vi "LSMcontroller_v57.vi"() -> ()   [LabVIEW 2015] (continued)
                      frame "X-Y Image", Default {
                        n4025 = local read "Sampling rate"() -> (w685:dbl)
                      }
                      frame "Timetrace" {
                        n4026 = local read "srateAODOtt"() -> (w686:dbl)
                      }
                    }
                    n4027 = call "waveformsAObuffer.vi"("command"="get") -> ("AO wf out"=w684:waveform(dbl)[])  [unwired: 1 in]
                    n4028 = Build Array (concatenate)(w671, w669) -> (w675:digitalwaveform[])
                    n4029 = call "correctwaveformsizetemp.vi"("new sampling frequency (Hz)"=w665, "start"=FALSE, "reference waveforms to"=w676, "Analog waveforms in"=w684, "stop"=FALSE, "Digital waveforms in"=w675) -> ("analog wf out"=w679:waveform(dbl)[], "Digital wf out"=w677:digitalwaveform[], "measpoints"=w667:i32)
                    n4030 = local write "Analog Lines Plot"(w679) -> ()
                    n4031 = call "GetNumCamFramesv2.vi"("Digital Waveform Graph"=w677) -> ("Numeric"=w678:i32)  [unwired: 10 in]
                    n4032 = local write "Digital Lines Plot"(w677) -> ()
                    n4033 = call "waveformsAObuffer.vi"("AO wf in"=w679, "command"="set") -> ()  [unwired: 1 out]
                    n4034 = call "waveformsDObuffer.vi"("DO wf in"=w677, "command"="set") -> ()  [unwired: 1 out]
                    n4035 = local write "Total Camera Frames"(w678) -> ()
                    n4036 = local read "wavdet"() -> (w668:bool)
                    n4037 = case shown="True" w668 {
                      tunnel: w667 -> [_ w687]
                      frame False {
                      }
                      frame True {
                        n4038 = local write "# of frames"(w687) -> ()
                      }
                    }
                  }
                  frame #7 {
                    w693 = FALSE ("addAO")
                    n4039 = local read "finite samples"() -> (w694:bool)
                    n4040 = local read "continuous"() -> (w695:bool)
                    n4041 = local read "wavdet"() -> (w696:bool)
                    n4042 = call "2pparameters.vi"("command"="get") -> ("params out"=w699:T12)  [unwired: 1 in]
                    n4043 = Bundle By Name(cluster=w699, "finite"=w694, "cont"=w695, "wavdet"=w696) -> (w697:T12)
                    n4044 = call "2pparameters.vi"("Params in"=w697, "command"="set") -> ()  [unwired: 1 out]
                    n4045 = local write "addDO"(w693) -> ()
                    n4046 = property on="Add DO wave" class="Bool (strict)"("Val(Sgnl)"=w693) -> ()  [unwired: 2 in, 2 out]
                  }
                }
              }
            }
          }
          event "DO channels": Value Change {
            n4047 = event-data() -> ()  [unwired: 1 in, 6 out]
            n4048 = local read "DO channels"() -> (w703:u16)
            n4049 = call "2pparameters.vi"("command"="get") -> ("params out"=w705:T12)  [unwired: 1 in]
            n4050 = Unbundle By Name(w705) -> ("aDO"=w704:u32[])
            n4051 = Search 1D Array(1D array=w704, element=w703) -> (index of element=w702:i32)  [unwired: 1 in]
            n4052 = Equal?(x=w702, y=-1.0) -> (x = y?=w701:bool)
            n4053 = case shown="False" w701 {
              tunnel: w702 -> [w720 _]
              frame False {
                n4054 = call "waveformparamsv2.vi"("command"="get") -> ("Params out"=w715:T16)  [unwired: 4 in, 2 out]
                n4055 = Unbundle By Name(w715) -> ("DO parameters"=w713:T19)
                n4056 = Index Array(array=w713, index=w720) -> (element=w719:T20)
                n4057 = Unbundle By Name(w719) -> ("Digital DC (%)"=w718:dbl, "Digital phase"=w717:dbl, "Digital Freq (Hz)"=w716:dbl, "Sampling frequency (Hz)"=w708:dbl, "Digital time offset (s)"=w712:dbl, "padding value"=w711:dbl, "matlab wave file"=w710:path, "DOtab"=w709:dbl)
                n4058 = local write "Build digital waveform tabs"(w709) -> ()
                n4059 = local write "Digital DC (%)"(w718) -> ()
                n4060 = local write "Matlab waveform path DO"(w710) -> ()
                n4061 = local write "Digital time offset (s)"(w712) -> ()
                n4062 = local write "Matlab padding value DO"(w711) -> ()
                n4063 = local write "Digital padding value"(w711) -> ()
                n4064 = local write "Sampling rate \ncurrent wf"(w708) -> ()
                n4065 = local write "Digital Freq (Hz)"(w716) -> ()
                n4066 = local write "Digital phase (s)"(w717) -> ()
              }
              frame True {
              }
            }
          }
          event "Rem DO wave": Value Change {
            n4067 = event-data() -> ("NewVal"=w721:bool)  [unwired: 1 in, 5 out]
            n4068 = case shown="True" w721 {
              frame False {
              }
              frame True {
                n4069 = stacked-sequence {
                  seq-local: [_ _ w827 _ _ _ _] -> [_ _ _ _ w846 w857 _]
                  frame #0 {
                    n4070 = local read "Measurement"() -> (w722:T5)
                    n4071 = case shown="\"linescan\"" w722 {
                      frame "X-Y-t movie", Default {
                        n4072 = local read "avpp"() -> (w743:i32)
                        n4073 = local read "Angle ref"() -> (w742:dbl)
                        n4074 = local read "ROI Type"() -> (w741:u16)
                        n4075 = local read "xpixels ref"() -> (w738:i32)
                        n4076 = local read "Vx-min ref"() -> (w737:dbl)
                        n4077 = local read "Vx-max ref"() -> (w736:dbl)
                        n4078 = local read "ypixels ref"() -> (w734:i32)
                        n4079 = local read "Vy-min ref"() -> (w735:dbl)
                        n4080 = local read "Vy-max ref"() -> (w731:dbl)
                        n4081 = local read "Sampling rate"() -> (w725:dbl)
                        n4082 = local read "finite samples"() -> (w726:bool)
                        n4083 = local read "continuous"() -> (w729:bool)
                        n4084 = local read "wavdet"() -> (w730:bool)
                        n4085 = local read "# of frames"() -> (w728:i32)
                        n4086 = local read "maxbufferAI"() -> (w727:i32)
                        n4087 = local read "Override AI buffer"() -> (w723:bool)
                        n4088 = call "2pparameters.vi"("command"="get") -> ("params out"=w740:T12)  [unwired: 1 in]
                        n4089 = Bundle By Name(cluster=w740, "type"="X-Y-t movie", "avpp"=w743, "Angle Img"=w742, "Xpixels Img"=w738, "Vx-min Img"=w737, "VX-max Img"=w736, "Ypixels Img"=w734, "Vy-min Img"=w735, "Vy-max Img"=w731, "srate"=w725, "srate Img"=w725, "finite"=w726, "cont"=w729, "wavdet"=w730, "measpoints"=w728, "maxbufferAI"=w727, "Drawing Mode"=w741, "Vz-reset"=0.0, "AIoverride"=w723) -> (w732:T12)
                        n4090 = call "2pparameters.vi"("Params in"=w732, "command"="set") -> ()  [unwired: 1 out]
                      }
                      frame "X-Y-Z stack" {
                        n4091 = call "2pparameters.vi"("command"="get") -> ("params out"=w747:T12)  [unwired: 1 in]
                        n4092 = Bundle By Name(cluster=w747, "type"="X-Y-Z stack") -> (w745:T12)
                        n4093 = call "2pparameters.vi"("Params in"=w745, "command"="set") -> ()  [unwired: 1 out]
                      }
                      frame "Lifetime (scan)" {
                        n4094 = call "2pparameters.vi"("command"="get") -> ("params out"=w752:T12)  [unwired: 1 in]
                        n4095 = Bundle By Name(cluster=w752, "type"="Lifetime (scan)") -> (w750:T12)
                        n4096 = call "2pparameters.vi"("Params in"=w750, "command"="set") -> ()  [unwired: 1 out]
                      }
                      frame "Lifetime (contour)" {
                        n4097 = local read "Vy-min draw"() -> (w762:dbl)
                        n4098 = local read "Vy-max draw"() -> (w761:dbl)
                        n4099 = local read "Vx-min draw"() -> (w764:dbl)
                        n4100 = local read "Vx-max draw"() -> (w763:dbl)
                        n4101 = local read "xpixels ref"() -> (w760:i32)
                        n4102 = local read "ypixels ref"() -> (w759:i32)
                        n4103 = local read "ROI Type"() -> (w758:u16)
                        n4104 = local read "srateAODOtt"() -> (w769:dbl)
                        n4105 = local read "# of frames"() -> (w774:i32)
                        n4106 = local read "refreshtime"() -> (w766:dbl)
                        n4107 = local read "Pel"() -> (w757:dbl)
                        n4108 = local read "bin"() -> (w772:dbl)
                        n4109 = local read "Override AI buffer"() -> (w755:bool)
                        n4110 = local read "finite samples"() -> (w781:bool)
                        n4111 = local read "srateAODOtt"() -> (w768:dbl)
                        n4112 = local read "srateAODOtt"() -> (w775:dbl)
                        n4113 = local read "continuous"() -> (w780:bool)
                        n4114 = local read "Angle ref"() -> (w765:dbl)
                        n4115 = local read "wavdet"() -> (w782:bool)
                        n4116 = local read "Vx-ref"() -> (w777:dbl)
                        n4117 = local read "Vy-ref"() -> (w779:dbl)
                        n4118 = local read "avpp"() -> (w778:i32)
                        n4119 = call "tt_timeandsamples.vi"("bin"=w772, "refreshtime"=w766, "srateAODOtt"=w769, "tot#ofsamples"=w774) -> ("refreshrate"=w770:dbl, "refreshbuffer"=w771:i32, "timetracecycles"=w776:i32)  [unwired: 5 in]
                        n4120 = local read "bin"() -> (w773:dbl)
                        n4121 = call "2pparameters.vi"("command"="get") -> ("params out"=w785:T12)  [unwired: 1 in]
                        n4122 = Bundle By Name(cluster=w785, "Drawing Mode"=w758, "measpoints"=w774, "tt_cycles"=w776, "refreshbuffer"=w771, "refreshrate"=w770, "Vx-ref"=w777, "Vy-ref"=w779, "srate"=w768, "finite"=w781, "cont"=w780, "wavdet"=w782, "avpp"=w778, "srateAODO"=w775, "bufferAI"=w771, "bin"=w773, "Angle Img"=w765, "Vxminref"=w764, "Vxmaxref"=w763, "Vyminref"=w762, "Vymaxref"=w761, "Xpixels Img"=w760, "Ypixels Img"=w759, "Pel"=w757, "Vz-reset"=0.0, "AIoverride"=w755, "type"="Lifetime (contour)") -> (w783:T12)
                        n4123 = Reciprocal(x=w770) -> (1/x=w767:dbl)
                        n4124 = local write "refreshtime"(w767) -> ()
                        n4125 = call "2pparameters.vi"("Params in"=w783, "command"="set") -> ()  [unwired: 1 out]
                      }
                      frame "X-Y-Z-t movie" {
                      }
                      frame "linescan" {
                      }
                      frame "Timetrace" {
                        n4126 = local read "Vy-min draw"() -> (w795:dbl)
                        n4127 = local read "Vy-max draw"() -> (w794:dbl)
                        n4128 = local read "Vx-min draw"() -> (w797:dbl)
                        n4129 = local read "Vx-max draw"() -> (w796:dbl)
                        n4130 = local read "xpixels ref"() -> (w793:i32)
                        n4131 = local read "ypixels ref"() -> (w792:i32)
                        n4132 = local read "ROI Type"() -> (w791:u16)
                        n4133 = local read "srateAODOtt"() -> (w802:dbl)
                        n4134 = local read "# of frames"() -> (w807:i32)
                        n4135 = local read "refreshtime"() -> (w799:dbl)
                        n4136 = local read "Pel"() -> (w790:dbl)
                        n4137 = local read "bin"() -> (w805:dbl)
                        n4138 = local read "Override AI buffer"() -> (w788:bool)
                        n4139 = local read "finite samples"() -> (w814:bool)
                        n4140 = local read "srateAODOtt"() -> (w801:dbl)
                        n4141 = local read "srateAODOtt"() -> (w808:dbl)
                        n4142 = local read "continuous"() -> (w813:bool)
                        n4143 = local read "Angle ref"() -> (w798:dbl)
                        n4144 = local read "wavdet"() -> (w815:bool)
                        n4145 = local read "Vx-ref"() -> (w810:dbl)
                        n4146 = local read "Vy-ref"() -> (w812:dbl)
                        n4147 = local read "avpp"() -> (w811:i32)
                        n4148 = call "tt_timeandsamples.vi"("bin"=w805, "refreshtime"=w799, "srateAODOtt"=w802, "tot#ofsamples"=w807) -> ("refreshrate"=w803:dbl, "refreshbuffer"=w804:i32, "timetracecycles"=w809:i32)  [unwired: 5 in]
                        n4149 = local read "bin"() -> (w806:dbl)
                        n4150 = call "2pparameters.vi"("command"="get") -> ("params out"=w818:T12)  [unwired: 1 in]
                        n4151 = Bundle By Name(cluster=w818, "Drawing Mode"=w791, "measpoints"=w807, "tt_cycles"=w809, "refreshbuffer"=w804, "refreshrate"=w803, "Vx-ref"=w810, "Vy-ref"=w812, "srate"=w801, "finite"=w814, "cont"=w813, "wavdet"=w815, "avpp"=w811, "srateAODO"=w808, "bufferAI"=w804, "bin"=w806, "Angle Img"=w798, "Vxminref"=w797, "Vxmaxref"=w796, "Vyminref"=w795, "Vymaxref"=w794, "Xpixels Img"=w793, "Ypixels Img"=w792, "Pel"=w790, "Vz-reset"=0.0, "AIoverride"=w788, "type"="Timetrace") -> (w816:T12)
                        n4152 = Reciprocal(x=w803) -> (1/x=w800:dbl)
                        n4153 = local write "refreshtime"(w800) -> ()
                        n4154 = call "2pparameters.vi"("Params in"=w816, "command"="set") -> ()  [unwired: 1 out]
                      }
                      frame "Lifetime (point)" {
                      }
                    }
                  }
                  frame #1 {
                    w821 = FALSE ("wavdet")
                    n4155 = call "2pparameters.vi"("command"="get") -> ("params out"=w825:T12)  [unwired: 1 in]
                    n4156 = Bundle By Name(cluster=w825, "finite"=w821, "cont"=w821, "wavdet"=TRUE) -> (w822:T12)
                    n4157 = call "2pparameters.vi"("Params in"=w822, "command"="set") -> ()  [unwired: 1 out]
                  }
                  frame #2 {
                    n4158 = local read "DO channels"() -> (w833:u16)
                    n4159 = call "2pparameters.vi"("command"="get") -> ("params out"=w831:T12)  [unwired: 1 in]
                    n4160 = in-place {
                      in-place-border: w833 -> [w838]
                      in-place-border: [w835] -> w828
                      in-place-border: [w834] -> w827
                      n4161 = in-place-cluster #52(w831) -> ("aDO"=w837:u32[])
                      n4162 = call "remove channel from active arrayv2.vi"("line array in"=w837, "line to remove"=w838) -> ("line array out"=w836:u32[], "removal"=w835:bool, "index"=w834:i32)
                      n4163 = in-place-cluster #52("aDO"=w836) -> (w829:T12)
                    }
                    n4164 = local write "remDO"(w828) -> ()
                    n4165 = call "2pparameters.vi"("Params in"=w829, "command"="set") -> ()  [unwired: 1 out]
                  }
                  frame #3 {
                    n4166 = local read "remDO"() -> (w839:bool)
                    n4167 = case shown="True" w839 {
                      frame False {
                      }
                      frame True {
                        n4168 = call "Used AO lines.vi"() -> ("used AO names"=w843:string[], "used AO lines"=w845:tag[])  [unwired: 2 in]
                        n4169 = local write "Analog Used Lines"(w845) -> ()
                        n4170 = local write "Analog Used Names"(w843) -> ()
                        n4171 = call "Used DO lines.vi"() -> ("used DO names"=w841:string[], "used DO lines"=w840:tag[])  [unwired: 2 in]
                        n4172 = control-ref of="Analog Lines Plot"() -> (w844:refnum<vi>)
                        n4173 = control-ref of="Digital Lines Plot"() -> (w842:refnum<vi>)
                        n4174 = local write "Digital Used Lines"(w840) -> ()
                        n4175 = local write "Digital Used Names"(w841) -> ()
                        n4176 = call "prepAOWaveplot.vi"("WaveformGraph in"=w844, "Analog Used Names"=w843) -> ()  [unwired: 1 in]
                        n4177 = call "prepDOWaveplot.vi"("DigitalGraph in"=w842, "used DO names"=w841) -> ()  [unwired: 1 in]
                      }
                    }
                  }
                  frame #4 {
                    n4178 = local read "remDO"() -> (w847:bool)
                    n4179 = case shown="True" w847 {
                      tunnel: w846 -> [_ w848]
                      frame False {
                      }
                      frame True {
                        n4180 = call "waveformparamsv2.vi"("command"="rem DO", "index"=w848) -> ()  [unwired: 3 in, 3 out]
                      }
                    }
                  }
                  frame #5 {
                    n4181 = local read "Meastab"() -> (w853:enum32{"X-Y Image", "Linescan", "Timetrace"})
                    n4182 = property on="refwf" class="Ring (strict)"() -> ("RingText.Text"=w860:string)  [unwired: 2 in, 2 out]
                    n4183 = call "waveformsDObuffer.vi"("command"="get") -> ("DO wf out"=w859:digitalwaveform[])  [unwired: 1 in]
                    n4184 = case shown="\"Timetrace\"" w853 {
                      tunnel: [w869 w870] -> w852
                      frame "X-Y Image", Default {
                        n4185 = local read "Sampling rate"() -> (w869:dbl)
                      }
                      frame "Timetrace" {
                        n4186 = local read "srateAODOtt"() -> (w870:dbl)
                      }
                    }
                    n4187 = call "waveformsAObuffer.vi"("command"="get") -> ("AO wf out"=w868:waveform(dbl)[])  [unwired: 1 in]
                    n4188 = Delete From Array(array=w859, length=1, index=w857) -> (array with subset deleted=w856:digitalwaveform[])  [unwired: 1 out]
                    n4189 = call "correctwaveformsizetemp.vi"("new sampling frequency (Hz)"=w852, "start"=FALSE, "reference waveforms to"=w860, "Analog waveforms in"=w868, "stop"=FALSE, "Digital waveforms in"=w856) -> ("analog wf out"=w863:waveform(dbl)[], "Digital wf out"=w861:digitalwaveform[], "measpoints"=w854:i32)
                    n4190 = local read "wavdet"() -> (w855:bool)
                    n4191 = call "waveformsAObuffer.vi"("AO wf in"=w863, "command"="set") -> ()  [unwired: 1 out]
                    n4192 = call "waveformsDObuffer.vi"("DO wf in"=w861, "command"="set") -> ()  [unwired: 1 out]
                    n4193 = local write "Analog Lines Plot"(w863) -> ()
                    n4194 = local write "Digital Lines Plot"(w861) -> ()
                    n4195 = call "GetNumCamFramesv2.vi"("Digital Waveform Graph"=w861) -> ("Numeric"=w862:i32)  [unwired: 10 in]
                    n4196 = case shown="True" w855 {
                      tunnel: w854 -> [_ w871]
                      frame False {
                      }
                      frame True {
                        n4197 = local write "# of frames"(w871) -> ()
                      }
                    }
                    n4198 = local write "Total Camera Frames"(w862) -> ()
                  }
                  frame #6 {
                    w872 = FALSE ("addAO")
                    n4199 = local read "finite samples"() -> (w873:bool)
                    n4200 = local read "continuous"() -> (w874:bool)
                    n4201 = local read "wavdet"() -> (w875:bool)
                    n4202 = local write "remDO"(w872) -> ()
                    n4203 = call "2pparameters.vi"("command"="get") -> ("params out"=w878:T12)  [unwired: 1 in]
                    n4204 = Bundle By Name(cluster=w878, "finite"=w873, "cont"=w874, "wavdet"=w875) -> (w876:T12)
                    n4205 = property on="Rem DO wave" class="Bool (strict)"("Val(Sgnl)"=w872) -> ()  [unwired: 2 in, 2 out]
                    n4206 = call "2pparameters.vi"("Params in"=w876, "command"="set") -> ()  [unwired: 1 out]
                  }
                }
              }
            }
          }
          event "Digital phase (s)", "Digital DC (%)", "Digital Freq (Hz)", "Digital padding value", "Digital time offset (s)": Value Change {
            n4207 = event-data() -> ()  [unwired: 1 in, 6 out]
            n4208 = stacked-sequence {
              seq-local: [_ _ w986 _ _] -> [_ _ _ w1003 _]
              seq-local: [_ _ w985 _ _] -> [_ _ _ w1002 _]
              frame #0 {
                n4209 = local read "Measurement"() -> (w880:T5)
                n4210 = case shown="\"X-Y-t movie\", Default" w880 {
                  frame "X-Y-t movie", Default {
                    n4211 = local read "avpp"() -> (w901:i32)
                    n4212 = local read "Angle ref"() -> (w900:dbl)
                    n4213 = local read "ROI Type"() -> (w899:u16)
                    n4214 = local read "xpixels ref"() -> (w896:i32)
                    n4215 = local read "Vx-min ref"() -> (w895:dbl)
                    n4216 = local read "Vx-max ref"() -> (w894:dbl)
                    n4217 = local read "ypixels ref"() -> (w892:i32)
                    n4218 = local read "Vy-min ref"() -> (w893:dbl)
                    n4219 = local read "Vy-max ref"() -> (w889:dbl)
                    n4220 = local read "Sampling rate"() -> (w883:dbl)
                    n4221 = local read "finite samples"() -> (w884:bool)
                    n4222 = local read "continuous"() -> (w887:bool)
                    n4223 = local read "wavdet"() -> (w888:bool)
                    n4224 = local read "# of frames"() -> (w886:i32)
                    n4225 = local read "maxbufferAI"() -> (w885:i32)
                    n4226 = local read "Override AI buffer"() -> (w881:bool)
                    n4227 = call "2pparameters.vi"("command"="get") -> ("params out"=w898:T12)  [unwired: 1 in]
                    n4228 = Bundle By Name(cluster=w898, "type"="X-Y-t movie", "avpp"=w901, "Angle Img"=w900, "Xpixels Img"=w896, "Vx-min Img"=w895, "VX-max Img"=w894, "Ypixels Img"=w892, "Vy-min Img"=w893, "Vy-max Img"=w889, "srate"=w883, "srate Img"=w883, "finite"=w884, "cont"=w887, "wavdet"=w888, "measpoints"=w886, "maxbufferAI"=w885, "Drawing Mode"=w899, "Vz-reset"=0.0, "AIoverride"=w881) -> (w890:T12)
                    n4229 = call "2pparameters.vi"("Params in"=w890, "command"="set") -> ()  [unwired: 1 out]
                  }
                  frame "X-Y-Z stack" {
                    n4230 = call "2pparameters.vi"("command"="get") -> ("params out"=w905:T12)  [unwired: 1 in]
                    n4231 = Bundle By Name(cluster=w905, "type"="X-Y-Z stack") -> (w903:T12)
                    n4232 = call "2pparameters.vi"("Params in"=w903, "command"="set") -> ()  [unwired: 1 out]
                  }
                  frame "Lifetime (scan)" {
                    n4233 = call "2pparameters.vi"("command"="get") -> ("params out"=w910:T12)  [unwired: 1 in]
                    n4234 = Bundle By Name(cluster=w910, "type"="Lifetime (scan)") -> (w908:T12)
                    n4235 = call "2pparameters.vi"("Params in"=w908, "command"="set") -> ()  [unwired: 1 out]
                  }
                  frame "Lifetime (contour)" {
                    n4236 = local read "Vy-min draw"() -> (w920:dbl)
                    n4237 = local read "Vy-max draw"() -> (w919:dbl)
                    n4238 = local read "Vx-min draw"() -> (w922:dbl)
                    n4239 = local read "Vx-max draw"() -> (w921:dbl)
                    n4240 = local read "xpixels ref"() -> (w918:i32)
                    n4241 = local read "ypixels ref"() -> (w917:i32)
                    n4242 = local read "ROI Type"() -> (w916:u16)
                    n4243 = local read "srateAODOtt"() -> (w927:dbl)
                    n4244 = local read "# of frames"() -> (w932:i32)
                    n4245 = local read "refreshtime"() -> (w924:dbl)
                    n4246 = local read "Pel"() -> (w915:dbl)
                    n4247 = local read "bin"() -> (w930:dbl)
                    n4248 = local read "Override AI buffer"() -> (w913:bool)
                    n4249 = local read "finite samples"() -> (w939:bool)
                    n4250 = local read "srateAODOtt"() -> (w926:dbl)
                    n4251 = local read "srateAODOtt"() -> (w933:dbl)
                    n4252 = local read "continuous"() -> (w938:bool)
                    n4253 = local read "Angle ref"() -> (w923:dbl)
                    n4254 = local read "wavdet"() -> (w940:bool)
                    n4255 = local read "Vx-ref"() -> (w935:dbl)
                    n4256 = local read "Vy-ref"() -> (w937:dbl)
                    n4257 = local read "avpp"() -> (w936:i32)
                    n4258 = call "tt_timeandsamples.vi"("bin"=w930, "refreshtime"=w924, "srateAODOtt"=w927, "tot#ofsamples"=w932) -> ("refreshrate"=w928:dbl, "refreshbuffer"=w929:i32, "timetracecycles"=w934:i32)  [unwired: 5 in]
                    n4259 = local read "bin"() -> (w931:dbl)
                    n4260 = call "2pparameters.vi"("command"="get") -> ("params out"=w943:T12)  [unwired: 1 in]
                    n4261 = Bundle By Name(cluster=w943, "Drawing Mode"=w916, "measpoints"=w932, "tt_cycles"=w934, "refreshbuffer"=w929, "refreshrate"=w928, "Vx-ref"=w935, "Vy-ref"=w937, "srate"=w926, "finite"=w939, "cont"=w938, "wavdet"=w940, "avpp"=w936, "srateAODO"=w933, "bufferAI"=w929, "bin"=w931, "Angle Img"=w923, "Vxminref"=w922, "Vxmaxref"=w921, "Vyminref"=w920, "Vymaxref"=w919, "Xpixels Img"=w918, "Ypixels Img"=w917, "Pel"=w915, "Vz-reset"=0.0, "AIoverride"=w913, "type"="Lifetime (contour)") -> (w941:T12)
                    n4262 = Reciprocal(x=w928) -> (1/x=w925:dbl)
                    n4263 = local write "refreshtime"(w925) -> ()
                    n4264 = call "2pparameters.vi"("Params in"=w941, "command"="set") -> ()  [unwired: 1 out]
                  }
                  frame "X-Y-Z-t movie" {
                  }
                  frame "linescan" {
                  }
                  frame "Timetrace" {
                    n4265 = local read "Vy-min draw"() -> (w953:dbl)
                    n4266 = local read "Vy-max draw"() -> (w952:dbl)
                    n4267 = local read "Vx-min draw"() -> (w955:dbl)
                    n4268 = local read "Vx-max draw"() -> (w954:dbl)
                    n4269 = local read "xpixels ref"() -> (w951:i32)
                    n4270 = local read "ypixels ref"() -> (w950:i32)
                    n4271 = local read "ROI Type"() -> (w949:u16)
                    n4272 = local read "srateAODOtt"() -> (w960:dbl)
                    n4273 = local read "# of frames"() -> (w965:i32)
                    n4274 = local read "refreshtime"() -> (w957:dbl)
                    n4275 = local read "Pel"() -> (w948:dbl)
                    n4276 = local read "bin"() -> (w963:dbl)
                    n4277 = local read "Override AI buffer"() -> (w946:bool)
                    n4278 = local read "finite samples"() -> (w972:bool)
                    n4279 = local read "srateAODOtt"() -> (w959:dbl)
                    n4280 = local read "srateAODOtt"() -> (w966:dbl)
                    n4281 = local read "continuous"() -> (w971:bool)
                    n4282 = local read "Angle ref"() -> (w956:dbl)
                    n4283 = local read "wavdet"() -> (w973:bool)
                    n4284 = local read "Vx-ref"() -> (w968:dbl)
                    n4285 = local read "Vy-ref"() -> (w970:dbl)
                    n4286 = local read "avpp"() -> (w969:i32)
                    n4287 = call "tt_timeandsamples.vi"("bin"=w963, "refreshtime"=w957, "srateAODOtt"=w960, "tot#ofsamples"=w965) -> ("refreshrate"=w961:dbl, "refreshbuffer"=w962:i32, "timetracecycles"=w967:i32)  [unwired: 5 in]
                    n4288 = local read "bin"() -> (w964:dbl)
                    n4289 = call "2pparameters.vi"("command"="get") -> ("params out"=w976:T12)  [unwired: 1 in]
                    n4290 = Bundle By Name(cluster=w976, "Drawing Mode"=w949, "measpoints"=w965, "tt_cycles"=w967, "refreshbuffer"=w962, "refreshrate"=w961, "Vx-ref"=w968, "Vy-ref"=w970, "srate"=w959, "finite"=w972, "cont"=w971, "wavdet"=w973, "avpp"=w969, "srateAODO"=w966, "bufferAI"=w962, "bin"=w964, "Angle Img"=w956, "Vxminref"=w955, "Vxmaxref"=w954, "Vyminref"=w953, "Vymaxref"=w952, "Xpixels Img"=w951, "Ypixels Img"=w950, "Pel"=w948, "Vz-reset"=0.0, "AIoverride"=w946, "type"="Timetrace") -> (w974:T12)
                    n4291 = Reciprocal(x=w961) -> (1/x=w958:dbl)
                    n4292 = local write "refreshtime"(w958) -> ()
                    n4293 = call "2pparameters.vi"("Params in"=w974, "command"="set") -> ()  [unwired: 1 out]
                  }
                  frame "Lifetime (point)" {
                  }
                }
              }
              frame #1 {
                w979 = FALSE ("wavdet")
                n4294 = call "2pparameters.vi"("command"="get") -> ("params out"=w983:T12)  [unwired: 1 in]
                n4295 = Bundle By Name(cluster=w983, "finite"=w979, "cont"=w979, "wavdet"=TRUE) -> (w980:T12)
                n4296 = call "2pparameters.vi"("Params in"=w980, "command"="set") -> ()  [unwired: 1 out]
              }
              frame #2 {
                n4297 = local read "DO channels"() -> (w988:u16)
                n4298 = call "2pparameters.vi"("command"="get") -> ("params out"=w990:T12)  [unwired: 1 in]
                n4299 = Unbundle By Name(w990) -> ("aDO"=w989:u32[])
                n4300 = Search 1D Array(1D array=w989, element=w988) -> (index of element=w986:i32)  [unwired: 1 in]
                n4301 = Greater?(x=w986, y=-1) -> (0:w985:bool)
                n4302 = case shown="True" w985 {
                  tunnel: w986 -> [_ w999]
                  frame False {
                  }
                  frame True {
                    n4303 = local read "Meastab"() -> (w993:enum32{"X-Y Image", "Linescan", "Timetrace"})
                    n4304 = local read "Digital padding value"() -> (w994:dbl)
                    n4305 = local read "Digital time offset (s)"() -> (w995:dbl)
                    n4306 = case shown="\"Timetrace\"" w993 {
                      tunnel: [w1000 w1001] -> w992
                      frame "X-Y Image", Default {
                        n4307 = local read "Sampling rate"() -> (w1000:dbl)
                      }
                      frame "Timetrace" {
                        n4308 = local read "srateAODOtt"() -> (w1001:dbl)
                      }
                    }
                    n4309 = local read "Digital Freq (Hz)"() -> (w997:dbl)
                    n4310 = local read "Digital phase (s)"() -> (w996:dbl)
                    n4311 = local read "Digital DC (%)"() -> (w998:dbl)
                    n4312 = call "replace DO wf param.vi"("Digital Freq (Hz)"=w997, "Digital DC (%)"=w998, "Digital phase"=w996, "Sampling frequency (Hz)"=w992, "Digital time offset (s)"=w995, "index of DO wave"=w999, "padding value"=w994) -> ()  [unwired: 4 in]
                  }
                }
              }
              frame #3 {
                n4313 = case shown="True" w1002 {
                  tunnel: w1003 -> [_ w1010]
                  frame False {
                  }
                  frame True {
                    n4314 = local read "Meastab"() -> (w1007:enum32{"X-Y Image", "Linescan", "Timetrace"})
                    n4315 = call "waveformparamsv2.vi"("command"="get") -> ("Params out"=w1026:T16)  [unwired: 4 in, 2 out]
                    n4316 = Unbundle By Name(w1026) -> ("DO parameters"=w1025:T19)
                    n4317 = property on="refwf" class="Ring (strict)"() -> ("RingText.Text"=w1032:string)  [unwired: 2 in, 2 out]
                    n4318 = case shown="\"Timetrace\"" w1007 {
                      tunnel: [w1033 w1034] -> w1006
                      frame "X-Y Image", Default {
                        n4319 = local read "Sampling rate"() -> (w1033:dbl)
                      }
                      frame "Timetrace" {
                        n4320 = local read "srateAODOtt"() -> (w1034:dbl)
                      }
                    }
                    n4321 = call "waveformsAObuffer.vi"("command"="get") -> ("AO wf out"=w1030:waveform(dbl)[])  [unwired: 1 in]
                    n4322 = call "waveformsDObuffer.vi"("command"="get") -> ("DO wf out"=w1028:digitalwaveform[])  [unwired: 1 in]
                    n4323 = call "referfencesize.vi"("Digital waveforms in"=w1028, "Analog waveforms in"=w1030, "reference waveforms to"=w1032) -> ("number of samples"=w1023:i32)  [unwired: 2 in]
                    n4324 = Index Array(array=w1025, index=w1010) -> (element=w1024:T20)
                    n4325 = call "waveformsDObuffer.vi"("command"="get") -> ("DO wf out"=w1020:digitalwaveform[])  [unwired: 1 in]
                    n4326 = call "simple digital from wf params.vi"("waveform params"=w1024, "number of samples"=w1023) -> ("digital waveform"=w1022:digitalwaveform)
                    n4327 = property on="refwf" class="Ring (strict)"() -> ("RingText.Text"=w1012:string)  [unwired: 2 in, 2 out]
                    n4328 = Replace Array Subset(array=w1020, new element=w1022, index=w1010) -> (w1011:digitalwaveform[])
                    n4329 = call "waveformsAObuffer.vi"("command"="get") -> ("AO wf out"=w1019:waveform(dbl)[])  [unwired: 1 in]
                    n4330 = local read "wavdet"() -> (w1009:bool)
                    n4331 = call "correctwaveformsizetemp.vi"("new sampling frequency (Hz)"=w1006, "start"=FALSE, "reference waveforms to"=w1012, "Analog waveforms in"=w1019, "stop"=FALSE, "Digital waveforms in"=w1011) -> ("analog wf out"=w1015:waveform(dbl)[], "Digital wf out"=w1013:digitalwaveform[], "measpoints"=w1008:i32)
                    n4332 = local write "Analog Lines Plot"(w1015) -> ()
                    n4333 = call "GetNumCamFramesv2.vi"("Digital Waveform Graph"=w1013) -> ("Numeric"=w1014:i32)  [unwired: 10 in]
                    n4334 = local write "Digital Lines Plot"(w1013) -> ()
                    n4335 = case shown="True" w1009 {
                      tunnel: w1008 -> [_ w1035]
                      frame False {
                      }
                      frame True {
                        n4336 = local write "# of frames"(w1035) -> ()
                      }
                    }
                    n4337 = call "waveformsAObuffer.vi"("AO wf in"=w1015, "command"="set") -> ()  [unwired: 1 out]
                    n4338 = call "waveformsDObuffer.vi"("DO wf in"=w1013, "command"="set") -> ()  [unwired: 1 out]
                    n4339 = local write "Total Camera Frames"(w1014) -> ()
                  }
                }
              }
              frame #4 {
                n4340 = local read "finite samples"() -> (w1036:bool)
                n4341 = local read "continuous"() -> (w1037:bool)
                n4342 = local read "wavdet"() -> (w1038:bool)
                n4343 = call "2pparameters.vi"("command"="get") -> ("params out"=w1041:T12)  [unwired: 1 in]
                n4344 = Bundle By Name(cluster=w1041, "finite"=w1036, "cont"=w1037, "wavdet"=w1038) -> (w1039:T12)
                n4345 = call "2pparameters.vi"("Params in"=w1039, "command"="set") -> ()  [unwired: 1 out]
              }
            }
          }
          event "refwf": Value Change {
            n4346 = event-data() -> ()  [unwired: 1 in, 6 out]
            n4347 = stacked-sequence {
              frame #0 {
                n4348 = local read "Measurement"() -> (w1043:T5)
                n4349 = case shown="\"X-Y-t movie\", Default" w1043 {
                  frame "X-Y-t movie", Default {
                    n4350 = local read "avpp"() -> (w1064:i32)
                    n4351 = local read "Angle ref"() -> (w1063:dbl)
                    n4352 = local read "ROI Type"() -> (w1062:u16)
                    n4353 = local read "xpixels ref"() -> (w1059:i32)
                    n4354 = local read "Vx-min ref"() -> (w1058:dbl)
                    n4355 = local read "Vx-max ref"() -> (w1057:dbl)
                    n4356 = local read "ypixels ref"() -> (w1055:i32)
                    n4357 = local read "Vy-min ref"() -> (w1056:dbl)
                    n4358 = local read "Vy-max ref"() -> (w1052:dbl)
                    n4359 = local read "Sampling rate"() -> (w1046:dbl)
                    n4360 = local read "finite samples"() -> (w1047:bool)
                    n4361 = local read "continuous"() -> (w1050:bool)
                    n4362 = local read "wavdet"() -> (w1051:bool)
                    n4363 = local read "# of frames"() -> (w1049:i32)
                    n4364 = local read "maxbufferAI"() -> (w1048:i32)
                    n4365 = local read "Override AI buffer"() -> (w1044:bool)
                    n4366 = call "2pparameters.vi"("command"="get") -> ("params out"=w1061:T12)  [unwired: 1 in]
                    n4367 = Bundle By Name(cluster=w1061, "type"="X-Y-t movie", "avpp"=w1064, "Angle Img"=w1063, "Xpixels Img"=w1059, "Vx-min Img"=w1058, "VX-max Img"=w1057, "Ypixels Img"=w1055, "Vy-min Img"=w1056, "Vy-max Img"=w1052, "srate"=w1046, "srate Img"=w1046, "finite"=w1047, "cont"=w1050, "wavdet"=w1051, "measpoints"=w1049, "maxbufferAI"=w1048, "Drawing Mode"=w1062, "Vz-reset"=0.0, "AIoverride"=w1044) -> (w1053:T12)
                    n4368 = call "2pparameters.vi"("Params in"=w1053, "command"="set") -> ()  [unwired: 1 out]
                  }
                  frame "X-Y-Z stack" {
                    n4369 = call "2pparameters.vi"("command"="get") -> ("params out"=w1068:T12)  [unwired: 1 in]
                    n4370 = Bundle By Name(cluster=w1068, "type"="X-Y-Z stack") -> (w1066:T12)
                    n4371 = call "2pparameters.vi"("Params in"=w1066, "command"="set") -> ()  [unwired: 1 out]
                  }
                  frame "Lifetime (scan)" {
                    n4372 = call "2pparameters.vi"("command"="get") -> ("params out"=w1073:T12)  [unwired: 1 in]
                    n4373 = Bundle By Name(cluster=w1073, "type"="Lifetime (scan)") -> (w1071:T12)
                    n4374 = call "2pparameters.vi"("Params in"=w1071, "command"="set") -> ()  [unwired: 1 out]
                  }
                  frame "Lifetime (contour)" {
                    n4375 = local read "Vy-min draw"() -> (w1083:dbl)
                    n4376 = local read "Vy-max draw"() -> (w1082:dbl)
                    n4377 = local read "Vx-min draw"() -> (w1085:dbl)
                    n4378 = local read "Vx-max draw"() -> (w1084:dbl)
                    n4379 = local read "xpixels ref"() -> (w1081:i32)
                    n4380 = local read "ypixels ref"() -> (w1080:i32)
                    n4381 = local read "ROI Type"() -> (w1079:u16)
                    n4382 = local read "srateAODOtt"() -> (w1090:dbl)
                    n4383 = local read "# of frames"() -> (w1095:i32)
                    n4384 = local read "refreshtime"() -> (w1087:dbl)
                    n4385 = local read "Pel"() -> (w1078:dbl)
                    n4386 = local read "bin"() -> (w1093:dbl)
                    n4387 = local read "Override AI buffer"() -> (w1076:bool)
                    n4388 = local read "finite samples"() -> (w1102:bool)
                    n4389 = local read "srateAODOtt"() -> (w1089:dbl)
                    n4390 = local read "srateAODOtt"() -> (w1096:dbl)
                    n4391 = local read "continuous"() -> (w1101:bool)
                    n4392 = local read "Angle ref"() -> (w1086:dbl)
                    n4393 = local read "wavdet"() -> (w1103:bool)
                    n4394 = local read "Vx-ref"() -> (w1098:dbl)
                    n4395 = local read "Vy-ref"() -> (w1100:dbl)
                    n4396 = local read "avpp"() -> (w1099:i32)
                    n4397 = call "tt_timeandsamples.vi"("bin"=w1093, "refreshtime"=w1087, "srateAODOtt"=w1090, "tot#ofsamples"=w1095) -> ("refreshrate"=w1091:dbl, "refreshbuffer"=w1092:i32, "timetracecycles"=w1097:i32)  [unwired: 5 in]
                    n4398 = local read "bin"() -> (w1094:dbl)
                    n4399 = call "2pparameters.vi"("command"="get") -> ("params out"=w1106:T12)  [unwired: 1 in]
                    n4400 = Bundle By Name(cluster=w1106, "Drawing Mode"=w1079, "measpoints"=w1095, "tt_cycles"=w1097, "refreshbuffer"=w1092, "refreshrate"=w1091, "Vx-ref"=w1098, "Vy-ref"=w1100, "srate"=w1089, "finite"=w1102, "cont"=w1101, "wavdet"=w1103, "avpp"=w1099, "srateAODO"=w1096, "bufferAI"=w1092, "bin"=w1094, "Angle Img"=w1086, "Vxminref"=w1085, "Vxmaxref"=w1084, "Vyminref"=w1083, "Vymaxref"=w1082, "Xpixels Img"=w1081, "Ypixels Img"=w1080, "Pel"=w1078, "Vz-reset"=0.0, "AIoverride"=w1076, "type"="Lifetime (contour)") -> (w1104:T12)
                    n4401 = Reciprocal(x=w1091) -> (1/x=w1088:dbl)
                    n4402 = local write "refreshtime"(w1088) -> ()
                    n4403 = call "2pparameters.vi"("Params in"=w1104, "command"="set") -> ()  [unwired: 1 out]
                  }
                  frame "X-Y-Z-t movie" {
                  }
                  frame "linescan" {
                  }
                  frame "Timetrace" {
                    n4404 = local read "Vy-min draw"() -> (w1116:dbl)
                    n4405 = local read "Vy-max draw"() -> (w1115:dbl)
                    n4406 = local read "Vx-min draw"() -> (w1118:dbl)
                    n4407 = local read "Vx-max draw"() -> (w1117:dbl)
                    n4408 = local read "xpixels ref"() -> (w1114:i32)
                    n4409 = local read "ypixels ref"() -> (w1113:i32)
                    n4410 = local read "ROI Type"() -> (w1112:u16)
                    n4411 = local read "srateAODOtt"() -> (w1123:dbl)
                    n4412 = local read "# of frames"() -> (w1128:i32)
                    n4413 = local read "refreshtime"() -> (w1120:dbl)
                    n4414 = local read "Pel"() -> (w1111:dbl)
                    n4415 = local read "bin"() -> (w1126:dbl)
                    n4416 = local read "Override AI buffer"() -> (w1109:bool)
                    n4417 = local read "finite samples"() -> (w1135:bool)
                    n4418 = local read "srateAODOtt"() -> (w1122:dbl)
                    n4419 = local read "srateAODOtt"() -> (w1129:dbl)
                    n4420 = local read "continuous"() -> (w1134:bool)
                    n4421 = local read "Angle ref"() -> (w1119:dbl)
                    n4422 = local read "wavdet"() -> (w1136:bool)
                    n4423 = local read "Vx-ref"() -> (w1131:dbl)
                    n4424 = local read "Vy-ref"() -> (w1133:dbl)
                    n4425 = local read "avpp"() -> (w1132:i32)
                    n4426 = call "tt_timeandsamples.vi"("bin"=w1126, "refreshtime"=w1120, "srateAODOtt"=w1123, "tot#ofsamples"=w1128) -> ("refreshrate"=w1124:dbl, "refreshbuffer"=w1125:i32, "timetracecycles"=w1130:i32)  [unwired: 5 in]
                    n4427 = local read "bin"() -> (w1127:dbl)
                    n4428 = call "2pparameters.vi"("command"="get") -> ("params out"=w1139:T12)  [unwired: 1 in]
                    n4429 = Bundle By Name(cluster=w1139, "Drawing Mode"=w1112, "measpoints"=w1128, "tt_cycles"=w1130, "refreshbuffer"=w1125, "refreshrate"=w1124, "Vx-ref"=w1131, "Vy-ref"=w1133, "srate"=w1122, "finite"=w1135, "cont"=w1134, "wavdet"=w1136, "avpp"=w1132, "srateAODO"=w1129, "bufferAI"=w1125, "bin"=w1127, "Angle Img"=w1119, "Vxminref"=w1118, "Vxmaxref"=w1117, "Vyminref"=w1116, "Vymaxref"=w1115, "Xpixels Img"=w1114, "Ypixels Img"=w1113, "Pel"=w1111, "Vz-reset"=0.0, "AIoverride"=w1109, "type"="Timetrace") -> (w1137:T12)
                    n4430 = Reciprocal(x=w1124) -> (1/x=w1121:dbl)
                    n4431 = local write "refreshtime"(w1121) -> ()
                    n4432 = call "2pparameters.vi"("Params in"=w1137, "command"="set") -> ()  [unwired: 1 out]
                  }
                  frame "Lifetime (point)" {
                  }
                }
              }
              frame #1 {
                w1142 = FALSE ("wavdet")
                n4433 = call "2pparameters.vi"("command"="get") -> ("params out"=w1146:T12)  [unwired: 1 in]
                n4434 = Bundle By Name(cluster=w1146, "finite"=w1142, "cont"=w1142, "wavdet"=TRUE) -> (w1143:T12)
                n4435 = call "2pparameters.vi"("Params in"=w1143, "command"="set") -> ()  [unwired: 1 out]
              }
              frame #2 {
                n4436 = local read "Meastab"() -> (w1151:enum32{"X-Y Image", "Linescan", "Timetrace"})
                n4437 = property on="refwf" class="Ring (strict)"() -> ("RingText.Text"=w1154:string)  [unwired: 2 in, 2 out]
                n4438 = case shown="\"Timetrace\"" w1151 {
                  tunnel: [w1164 w1165] -> w1150
                  frame "X-Y Image", Default {
                    n4439 = local read "Sampling rate"() -> (w1164:dbl)
                  }
                  frame "Timetrace" {
                    n4440 = local read "srateAODOtt"() -> (w1165:dbl)
                  }
                }
                n4441 = call "waveformsAObuffer.vi"("command"="get") -> ("AO wf out"=w1163:waveform(dbl)[])  [unwired: 1 in]
                n4442 = local read "wavdet"() -> (w1153:bool)
                n4443 = call "waveformsDObuffer.vi"("command"="get") -> ("DO wf out"=w1159:digitalwaveform[])  [unwired: 1 in]
                n4444 = call "correctwaveformsizetemp.vi"("new sampling frequency (Hz)"=w1150, "start"=FALSE, "reference waveforms to"=w1154, "Analog waveforms in"=w1163, "stop"=FALSE, "Digital waveforms in"=w1159) -> ("analog wf out"=w1157:waveform(dbl)[], "Digital wf out"=w1155:digitalwaveform[], "measpoints"=w1152:i32)
                n4445 = local write "Analog Lines Plot"(w1157) -> ()
                n4446 = call "GetNumCamFramesv2.vi"("Digital Waveform Graph"=w1155) -> ("Numeric"=w1156:i32)  [unwired: 10 in]
                n4447 = local write "Digital Lines Plot"(w1155) -> ()
                n4448 = call "waveformsDObuffer.vi"("DO wf in"=w1155, "command"="set") -> ()  [unwired: 1 out]
                n4449 = call "waveformsAObuffer.vi"("AO wf in"=w1157, "command"="set") -> ()  [unwired: 1 out]
                n4450 = local write "Total Camera Frames"(w1156) -> ()
                n4451 = case shown="True" w1153 {
                  tunnel: w1152 -> [_ w1166]
                  frame False {
                  }
                  frame True {
                    n4452 = local write "# of frames"(w1166) -> ()
                  }
                }
              }
              frame #3 {
                n4453 = local read "finite samples"() -> (w1167:bool)
                n4454 = local read "continuous"() -> (w1168:bool)
                n4455 = local read "wavdet"() -> (w1169:bool)
                n4456 = call "2pparameters.vi"("command"="get") -> ("params out"=w1172:T12)  [unwired: 1 in]
                n4457 = Bundle By Name(cluster=w1172, "finite"=w1167, "cont"=w1168, "wavdet"=w1169) -> (w1170:T12)
                n4458 = call "2pparameters.vi"("Params in"=w1170, "command"="set") -> ()  [unwired: 1 out]
              }
            }
          }
          event "Start amplitude (V)", "Cycles", "Baseline (V)", "Step size (V)", "DC (%)", "Period (ms)", "Repeats", "Pulses", "phase shift (ms)": Value Change {
            n4459 = event-data() -> ()  [unwired: 1 in, 6 out]
            n4460 = stacked-sequence {
              seq-local: [_ _ w1280 _ _] -> [_ _ _ w1302 _]
              seq-local: [_ _ w1279 _ _] -> [_ _ _ w1301 _]
              frame #0 {
                n4461 = local read "Measurement"() -> (w1174:T5)
                n4462 = case shown="\"X-Y-t movie\", Default" w1174 {
                  frame "X-Y-t movie", Default {
                    n4463 = local read "avpp"() -> (w1195:i32)
                    n4464 = local read "Angle ref"() -> (w1194:dbl)
                    n4465 = local read "ROI Type"() -> (w1193:u16)
                    n4466 = local read "xpixels ref"() -> (w1190:i32)
                    n4467 = local read "Vx-min ref"() -> (w1189:dbl)
                    n4468 = local read "Vx-max ref"() -> (w1188:dbl)
                    n4469 = local read "ypixels ref"() -> (w1186:i32)
                    n4470 = local read "Vy-min ref"() -> (w1187:dbl)
                    n4471 = local read "Vy-max ref"() -> (w1183:dbl)
                    n4472 = local read "Sampling rate"() -> (w1177:dbl)
                    n4473 = local read "finite samples"() -> (w1178:bool)
                    n4474 = local read "continuous"() -> (w1181:bool)
                    n4475 = local read "wavdet"() -> (w1182:bool)
                    n4476 = local read "# of frames"() -> (w1180:i32)
                    n4477 = local read "maxbufferAI"() -> (w1179:i32)
                    n4478 = local read "Override AI buffer"() -> (w1175:bool)
                    n4479 = call "2pparameters.vi"("command"="get") -> ("params out"=w1192:T12)  [unwired: 1 in]
                    n4480 = Bundle By Name(cluster=w1192, "type"="X-Y-t movie", "avpp"=w1195, "Angle Img"=w1194, "Xpixels Img"=w1190, "Vx-min Img"=w1189, "VX-max Img"=w1188, "Ypixels Img"=w1186, "Vy-min Img"=w1187, "Vy-max Img"=w1183, "srate"=w1177, "srate Img"=w1177, "finite"=w1178, "cont"=w1181, "wavdet"=w1182, "measpoints"=w1180, "maxbufferAI"=w1179, "Drawing Mode"=w1193, "Vz-reset"=0.0, "AIoverride"=w1175) -> (w1184:T12)
                    n4481 = call "2pparameters.vi"("Params in"=w1184, "command"="set") -> ()  [unwired: 1 out]
                  }
                  frame "X-Y-Z stack" {
                    n4482 = call "2pparameters.vi"("command"="get") -> ("params out"=w1199:T12)  [unwired: 1 in]
                    n4483 = Bundle By Name(cluster=w1199, "type"="X-Y-Z stack") -> (w1197:T12)
                    n4484 = call "2pparameters.vi"("Params in"=w1197, "command"="set") -> ()  [unwired: 1 out]
                  }
                  frame "Lifetime (scan)" {
                    n4485 = call "2pparameters.vi"("command"="get") -> ("params out"=w1204:T12)  [unwired: 1 in]
                    n4486 = Bundle By Name(cluster=w1204, "type"="Lifetime (scan)") -> (w1202:T12)
                    n4487 = call "2pparameters.vi"("Params in"=w1202, "command"="set") -> ()  [unwired: 1 out]
                  }
                  frame "Lifetime (contour)" {
                    n4488 = local read "Vy-min draw"() -> (w1214:dbl)
                    n4489 = local read "Vy-max draw"() -> (w1213:dbl)
                    n4490 = local read "Vx-min draw"() -> (w1216:dbl)
                    n4491 = local read "Vx-max draw"() -> (w1215:dbl)
                    n4492 = local read "xpixels ref"() -> (w1212:i32)
                    n4493 = local read "ypixels ref"() -> (w1211:i32)
                    n4494 = local read "ROI Type"() -> (w1210:u16)
                    n4495 = local read "srateAODOtt"() -> (w1221:dbl)
                    n4496 = local read "# of frames"() -> (w1226:i32)
                    n4497 = local read "refreshtime"() -> (w1218:dbl)
                    n4498 = local read "Pel"() -> (w1209:dbl)
                    n4499 = local read "bin"() -> (w1224:dbl)
                    n4500 = local read "Override AI buffer"() -> (w1207:bool)
                    n4501 = local read "finite samples"() -> (w1233:bool)
                    n4502 = local read "srateAODOtt"() -> (w1220:dbl)
                    n4503 = local read "srateAODOtt"() -> (w1227:dbl)
                    n4504 = local read "continuous"() -> (w1232:bool)
                    n4505 = local read "Angle ref"() -> (w1217:dbl)
                    n4506 = local read "wavdet"() -> (w1234:bool)
                    n4507 = local read "Vx-ref"() -> (w1229:dbl)
                    n4508 = local read "Vy-ref"() -> (w1231:dbl)
                    n4509 = local read "avpp"() -> (w1230:i32)
                    n4510 = call "tt_timeandsamples.vi"("bin"=w1224, "refreshtime"=w1218, "srateAODOtt"=w1221, "tot#ofsamples"=w1226) -> ("refreshrate"=w1222:dbl, "refreshbuffer"=w1223:i32, "timetracecycles"=w1228:i32)  [unwired: 5 in]
                    n4511 = local read "bin"() -> (w1225:dbl)
                    n4512 = call "2pparameters.vi"("command"="get") -> ("params out"=w1237:T12)  [unwired: 1 in]
                    n4513 = Bundle By Name(cluster=w1237, "Drawing Mode"=w1210, "measpoints"=w1226, "tt_cycles"=w1228, "refreshbuffer"=w1223, "refreshrate"=w1222, "Vx-ref"=w1229, "Vy-ref"=w1231, "srate"=w1220, "finite"=w1233, "cont"=w1232, "wavdet"=w1234, "avpp"=w1230, "srateAODO"=w1227, "bufferAI"=w1223, "bin"=w1225, "Angle Img"=w1217, "Vxminref"=w1216, "Vxmaxref"=w1215, "Vyminref"=w1214, "Vymaxref"=w1213, "Xpixels Img"=w1212, "Ypixels Img"=w1211, "Pel"=w1209, "Vz-reset"=0.0, "AIoverride"=w1207, "type"="Lifetime (contour)") -> (w1235:T12)
                    n4514 = Reciprocal(x=w1222) -> (1/x=w1219:dbl)
                    n4515 = local write "refreshtime"(w1219) -> ()
                    n4516 = call "2pparameters.vi"("Params in"=w1235, "command"="set") -> ()  [unwired: 1 out]
                  }
                  frame "X-Y-Z-t movie" {
                  }
                  frame "linescan" {
                  }
                  frame "Timetrace" {
                    n4517 = local read "Vy-min draw"() -> (w1247:dbl)
                    n4518 = local read "Vy-max draw"() -> (w1246:dbl)
                    n4519 = local read "Vx-min draw"() -> (w1249:dbl)
                    n4520 = local read "Vx-max draw"() -> (w1248:dbl)
                    n4521 = local read "xpixels ref"() -> (w1245:i32)
                    n4522 = local read "ypixels ref"() -> (w1244:i32)
                    n4523 = local read "ROI Type"() -> (w1243:u16)
                    n4524 = local read "srateAODOtt"() -> (w1254:dbl)
                    n4525 = local read "# of frames"() -> (w1259:i32)
                    n4526 = local read "refreshtime"() -> (w1251:dbl)
                    n4527 = local read "Pel"() -> (w1242:dbl)
                    n4528 = local read "bin"() -> (w1257:dbl)
                    n4529 = local read "Override AI buffer"() -> (w1240:bool)
                    n4530 = local read "finite samples"() -> (w1266:bool)
                    n4531 = local read "srateAODOtt"() -> (w1253:dbl)
                    n4532 = local read "srateAODOtt"() -> (w1260:dbl)
                    n4533 = local read "continuous"() -> (w1265:bool)
                    n4534 = local read "Angle ref"() -> (w1250:dbl)
                    n4535 = local read "wavdet"() -> (w1267:bool)
                    n4536 = local read "Vx-ref"() -> (w1262:dbl)
                    n4537 = local read "Vy-ref"() -> (w1264:dbl)
                    n4538 = local read "avpp"() -> (w1263:i32)
                    n4539 = call "tt_timeandsamples.vi"("bin"=w1257, "refreshtime"=w1251, "srateAODOtt"=w1254, "tot#ofsamples"=w1259) -> ("refreshrate"=w1255:dbl, "refreshbuffer"=w1256:i32, "timetracecycles"=w1261:i32)  [unwired: 5 in]
                    n4540 = local read "bin"() -> (w1258:dbl)
                    n4541 = call "2pparameters.vi"("command"="get") -> ("params out"=w1270:T12)  [unwired: 1 in]
                    n4542 = Bundle By Name(cluster=w1270, "Drawing Mode"=w1243, "measpoints"=w1259, "tt_cycles"=w1261, "refreshbuffer"=w1256, "refreshrate"=w1255, "Vx-ref"=w1262, "Vy-ref"=w1264, "srate"=w1253, "finite"=w1266, "cont"=w1265, "wavdet"=w1267, "avpp"=w1263, "srateAODO"=w1260, "bufferAI"=w1256, "bin"=w1258, "Angle Img"=w1250, "Vxminref"=w1249, "Vxmaxref"=w1248, "Vyminref"=w1247, "Vymaxref"=w1246, "Xpixels Img"=w1245, "Ypixels Img"=w1244, "Pel"=w1242, "Vz-reset"=0.0, "AIoverride"=w1240, "type"="Timetrace") -> (w1268:T12)
                    n4543 = Reciprocal(x=w1255) -> (1/x=w1252:dbl)
                    n4544 = local write "refreshtime"(w1252) -> ()
                    n4545 = call "2pparameters.vi"("Params in"=w1268, "command"="set") -> ()  [unwired: 1 out]
                  }
                  frame "Lifetime (point)" {
                  }
                }
              }
              frame #1 {
                w1273 = FALSE ("wavdet")
                n4546 = call "2pparameters.vi"("command"="get") -> ("params out"=w1277:T12)  [unwired: 1 in]
                n4547 = Bundle By Name(cluster=w1277, "finite"=w1273, "cont"=w1273, "wavdet"=TRUE) -> (w1274:T12)
                n4548 = call "2pparameters.vi"("Params in"=w1274, "command"="set") -> ()  [unwired: 1 out]
              }
              frame #2 {
                n4549 = local read "AO channels"() -> (w1282:u32)
                n4550 = call "2pparameters.vi"("command"="get") -> ("params out"=w1284:T12)  [unwired: 1 in]
                n4551 = Unbundle By Name(w1284) -> ("aAO"=w1283:u32[])
                n4552 = Search 1D Array(1D array=w1283, element=w1282) -> (index of element=w1280:i32)  [unwired: 1 in]
                n4553 = Greater?(x=w1280, y=-1) -> (0:w1279:bool)
                n4554 = case shown="True" w1279 {
                  tunnel: w1280 -> [_ w1298]
                  frame False {
                  }
                  frame True {
                    n4555 = local read "Meastab"() -> (w1287:enum32{"X-Y Image", "Linescan", "Timetrace"})
                    n4556 = case shown="\"Timetrace\"" w1287 {
                      tunnel: [w1299 w1300] -> w1286
                      frame "X-Y Image", Default {
                        n4557 = local read "Sampling rate"() -> (w1299:dbl)
                      }
                      frame "Timetrace" {
                        n4558 = local read "srateAODOtt"() -> (w1300:dbl)
                      }
                    }
                    n4559 = local read "Start amplitude (V)"() -> (w1295:dbl)
                    n4560 = local read "phase shift (ms)"() -> (w1290:dbl)
                    n4561 = local read "Step size (V)"() -> (w1293:dbl)
                    n4562 = local read "Baseline (V)"() -> (w1294:dbl)
                    n4563 = local read "Period (ms)"() -> (w1291:dbl)
                    n4564 = local read "padding value"() -> (w1288:dbl)
                    n4565 = local read "Repeats"() -> (w1297:dbl)
                    n4566 = local read "Cycles"() -> (w1296:dbl)
                    n4567 = local read "DC (%)"() -> (w1292:dbl)
                    n4568 = local read "Pulses"() -> (w1289:dbl)
                    n4569 = call "replace AO square wf param.vi"("Baseline (V)"=w1294, "Start amplitude (V)"=w1295, "Cycles"=w1296, "Repeats"=w1297, "index of AO wave"=w1298, "Step size (V)"=w1293, "DC (%)"=w1292, "Sampling frequency (Hz)"=w1286, "Period (ms)"=w1291, "Cycle length (s)"=w1290, "Pulses"=w1289, "padding value"=w1288) -> ()  [unwired: 4 in]
                  }
                }
              }
              frame #3 {
                n4570 = case shown="True" w1301 {
                  tunnel: w1302 -> [_ w1310]
                  frame False {
                  }
                  frame True {
                    n4571 = call "waveformparamsv2.vi"("command"="get") -> ("Params out"=w1324:T16)  [unwired: 4 in, 2 out]
                    n4572 = Unbundle By Name(w1324) -> ("AO parameters"=w1323:T17)
                    n4573 = local read "Meastab"() -> (w1305:enum32{"X-Y Image", "Linescan", "Timetrace"})
                    n4574 = case shown="\"Timetrace\"" w1305 {
                      tunnel: [w1326 w1327] -> w1314
                      frame "X-Y Image", Default {
                        n4575 = local read "Sampling rate"() -> (w1326:dbl)
                      }
                      frame "Timetrace" {
                        n4576 = local read "srateAODOtt"() -> (w1327:dbl)
                      }
                    }
                    n4577 = Index Array(array=w1323, index=w1310) -> (element=w1312:T18)
                    n4578 = call "waveformsAObuffer.vi"("command"="get") -> ("AO wf out"=w1311:waveform(dbl)[])  [unwired: 1 in]
                    n4579 = call "generateRampedSquareWave_fromAOparameters.vi"("AO params"=w1312) -> ("Waveform"=w1309:waveform(dbl))  [unwired: 1 out]
                    n4580 = property on="refwf" class="Ring (strict)"() -> ("RingText.Text"=w1313:string)  [unwired: 2 in, 2 out]
                    n4581 = Replace Array Subset(array=w1311, new element=w1309, index=w1310) -> (w1308:waveform(dbl)[])
                    n4582 = call "waveformsDObuffer.vi"("command"="get") -> ("DO wf out"=w1319:digitalwaveform[])  [unwired: 1 in]
                    n4583 = call "correctwaveformsizetemp.vi"("new sampling frequency (Hz)"=w1314, "start"=FALSE, "reference waveforms to"=w1313, "Analog waveforms in"=w1308, "stop"=FALSE, "Digital waveforms in"=w1319) -> ("analog wf out"=w1317:waveform(dbl)[], "Digital wf out"=w1315:digitalwaveform[], "measpoints"=w1306:i32)
                    n4584 = local read "wavdet"() -> (w1307:bool)
                    n4585 = local write "Analog Lines Plot"(w1317) -> ()
                    n4586 = call "GetNumCamFramesv2.vi"("Digital Waveform Graph"=w1315) -> ("Numeric"=w1316:i32)  [unwired: 10 in]
                    n4587 = local write "Digital Lines Plot"(w1315) -> ()
                    n4588 = call "waveformsAObuffer.vi"("AO wf in"=w1317, "command"="set") -> ()  [unwired: 1 out]
                    n4589 = call "waveformsDObuffer.vi"("DO wf in"=w1315, "command"="set") -> ()  [unwired: 1 out]
                    n4590 = local write "Total Camera Frames"(w1316) -> ()
                    n4591 = case shown="True" w1307 {
                      tunnel: w1306 -> [_ w1328]
                      frame False {
                      }
                      frame True {
                        n4592 = local write "# of frames"(w1328) -> ()
                      }
                    }
                  }
                }
              }
              frame #4 {
                n4593 = local read "finite samples"() -> (w1329:bool)
                n4594 = local read "continuous"() -> (w1330:bool)
                n4595 = local read "wavdet"() -> (w1331:bool)
                n4596 = call "2pparameters.vi"("command"="get") -> ("params out"=w1334:T12)  [unwired: 1 in]
                n4597 = Bundle By Name(cluster=w1334, "finite"=w1329, "cont"=w1330, "wavdet"=w1331) -> (w1332:T12)
                n4598 = call "2pparameters.vi"("Params in"=w1332, "command"="set") -> ()  [unwired: 1 out]
              }
            }
          }
          event "Amplitude (V)", "Offset (V)", "Frequency", "Tri Repeats": Value Change {
            n4599 = event-data() -> ()  [unwired: 1 in, 6 out]
            n4600 = stacked-sequence {
              seq-local: [_ _ w1442 _ _] -> [_ _ _ w1460 _]
              seq-local: [_ _ w1441 _ _] -> [_ _ _ w1459 _]
              frame #0 {
                n4601 = local read "Measurement"() -> (w1336:T5)
                n4602 = case shown="\"X-Y-t movie\", Default" w1336 {
                  frame "X-Y-t movie", Default {
                    n4603 = local read "avpp"() -> (w1357:i32)
                    n4604 = local read "Angle ref"() -> (w1356:dbl)
                    n4605 = local read "ROI Type"() -> (w1355:u16)
                    n4606 = local read "xpixels ref"() -> (w1352:i32)
                    n4607 = local read "Vx-min ref"() -> (w1351:dbl)
                    n4608 = local read "Vx-max ref"() -> (w1350:dbl)
                    n4609 = local read "ypixels ref"() -> (w1348:i32)
                    n4610 = local read "Vy-min ref"() -> (w1349:dbl)
                    n4611 = local read "Vy-max ref"() -> (w1345:dbl)
                    n4612 = local read "Sampling rate"() -> (w1339:dbl)
                    n4613 = local read "finite samples"() -> (w1340:bool)
                    n4614 = local read "continuous"() -> (w1343:bool)
                    n4615 = local read "wavdet"() -> (w1344:bool)
                    n4616 = local read "# of frames"() -> (w1342:i32)
